vi "Create Data Queue.vi"() -> (0 "error out":errorcluster, 3 "queue out":refnum<queue>)   [LabVIEW 2020, in "Sensor910.lvclass"]
uses:
  Sensor910.lvclass
  Data.ctl
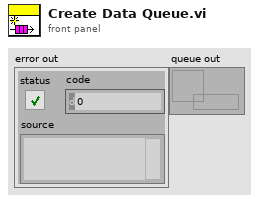
[diagram p1: front panel]
types:
  T1 = typedef "Sensor910.lvclass/Data.ctl" = cluster{"Connect":bool, "No Response":bool, "Data":sgl[]}
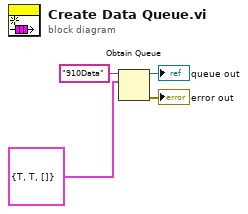
[diagram p0: block diagram]
diagram:
  n1 = Obtain Queue(name (unnamed)="910Data", element data type=T1 {"Connect"=TRUE, "No Response"=TRUE, "Data"=[]} ("Data")) -> (queue out=→"queue out":refnum<queue>, error out=→"error out":errorcluster)  [unwired: 3 in, 1 out]
